vi "Blocker Controller.vi"(11 "Blocker Toggle":bool) -> ()   [LabVIEW 2013]
uses:
  Systems/Blocker/Blocker.lvclass
  Robot Global Data.vi
  Commands/BL-Retract-Command/BL-Retract-Cmd.lvclass
  Commands/BL-Extend-Command/BL-Extend-Cmd.lvclass
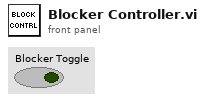
[diagram p1: front panel]
types:
  T1 = typedef "Semaphore RefNum" = refnum<k1>
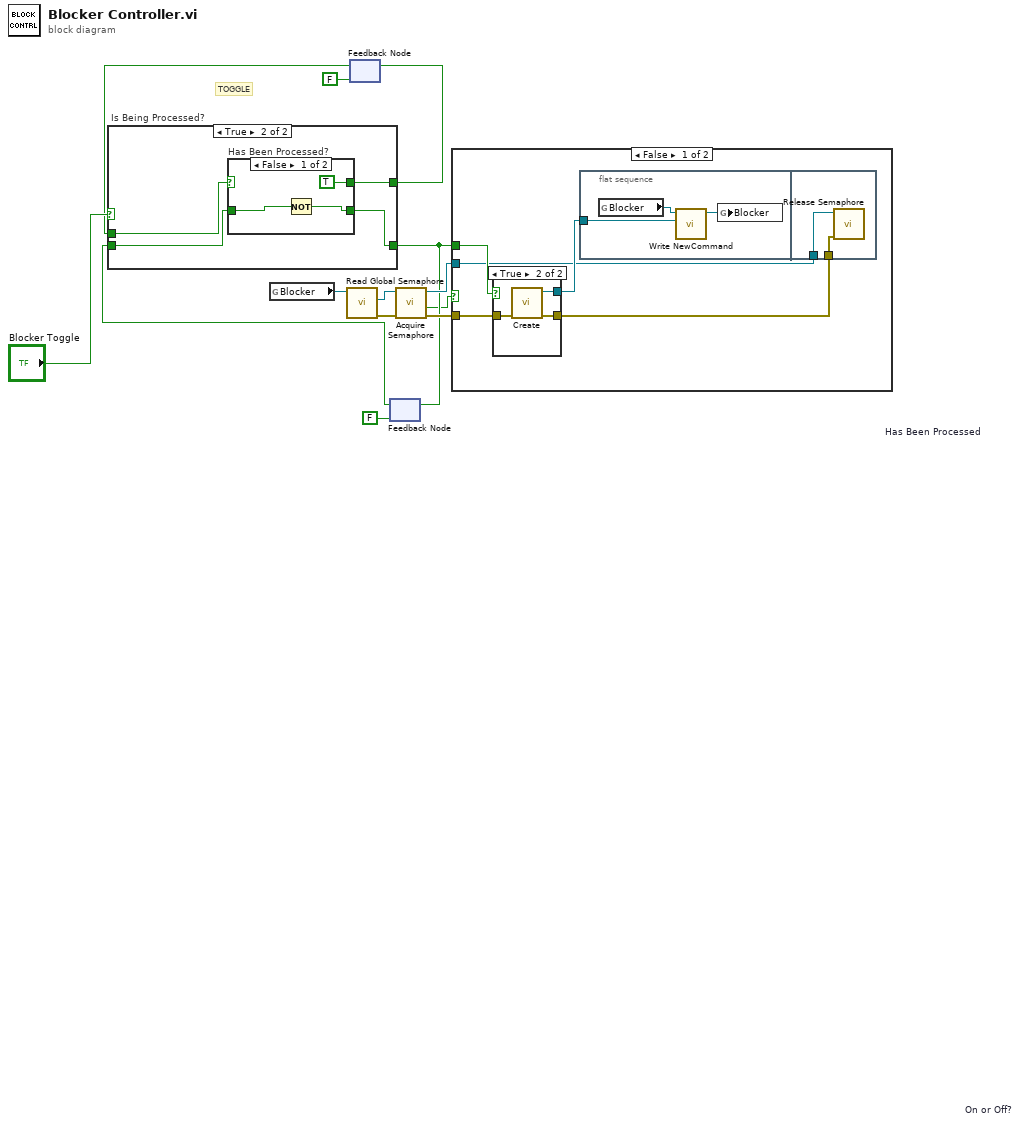
[diagram p0: block diagram]
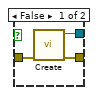
[diagram p2: hidden frame]
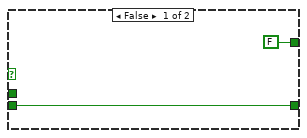
[diagram p4: hidden frame]
diagram:
  # "TOGGLE"
  n1 = global read "Robot Global Data.vi" "Blocker"() -> (w7:refnum<class "Blocker.lvclass">)
  n2 = call-dynamic "Read Global Semaphore.vi"("System in"=w7) -> ("error out"=w11:errorcluster, "semaphore"=w8:T1)  [unwired: 8 in, 1 out]
  n3 = feedback #1 "Has Been Processed"(FALSE) -> (w2:bool)
  n4 = feedback #2 "On or Off?"(FALSE) -> (w5:bool)
  n5 = case "Is Being Processed?" shown="True" "Blocker Toggle" {
    tunnel: w2 -> [_ w19]
    tunnel: [FALSE w18] -> w3
    tunnel: w5 -> [w14 w17]
    tunnel: [w14 w16] -> w10
    frame False {
    }
    frame True {
      n6 = case "Has Been Processed?" shown="False" w19 {
        selector: w19 -> [_ w24]
        tunnel: [TRUE w24] -> w18
        tunnel: w17 -> [w21 w23]
        tunnel: [w20 w23] -> w16
        frame False {
          n7 = Not(x=w21) -> (.not. x?=w20:bool)
        }
        frame True {
        }
      }
    }
  }
  n8 = feedback-in #1(w3) -> ()
  n9 = feedback-in #2(w10) -> ()
  n10 = call <vilib>:"Acquire Semaphore.vi"("error in (no error)"=w11, "semaphore"=w8) -> ("error out"=w12:errorcluster, "timed out"=w9:bool, "semaphore out"=w13:T1)  [unwired: 3 in]
  n11 = case shown="False" w9 {
    tunnel: w10 -> [w29 _]
    tunnel: w12 -> [w27 _]
    tunnel: w13 -> [w26 _]
    frame False {
      n12 = case shown="True" w29 {
        tunnel: [w32 w35] -> w28
        tunnel: w27 -> [w31 w34]
        tunnel: [w30 w33] -> w25
        frame False {
          n13 = call "Create.vi"("error in (no error)"=w31) -> ("error out"=w30:errorcluster, "BL-Retract-Cmd.lvclass"=w32:refnum<class "BL-Retract-Cmd.lvclass">)  [unwired: 9 in]
        }
        frame True {
          n14 = call "Create.vi"("error in (no error)"=w34) -> ("error out"=w33:errorcluster, "BL-Extend-Cmd out"=w35:refnum<class "BL-Extend-Cmd.lvclass">)  [unwired: 9 in]
        }
      }
      n15 = flat-sequence {
        tunnel: w28 -> [w36]
        tunnel: w26 -> [w40]
        tunnel: w25 -> [w39]
        frame #0 {
          n16 = global read "Robot Global Data.vi" "Blocker"() -> (w38:refnum<class "Blocker.lvclass">)
          n17 = call-dynamic "Write NewCommand.vi"("Command.lvclass"=w36, "System in"=w38) -> ("System out"=w37:refnum<class "Blocker.lvclass">)  [unwired: 8 in, 1 out]
          n18 = global write "Robot Global Data.vi" "Blocker"(w37) -> ()
        }
        frame #1 {
          n19 = call <vilib>:"Release Semaphore.vi"("error in (no error)"=w39, "semaphore"=w40) -> ()  [unwired: 4 in, 2 out]
        }
      }
    }
    frame True {
    }
  }
